vi "Remove.vi"(8 "Error In":errorcluster, 10 "IObserver":refnum<class "IObserver.lvclass">, 11 "reference in":refnum<class "CommunicationModule.lvclass">) -> (0 "Error Out":errorcluster, 3 "reference out":refnum<class "CommunicationModule.lvclass">)   [LabVIEW 2024, in "CommunicationModule.lvclass"]
doc: "Remove observer from the observer list"
uses:
  CommunicationModule.lvclass
  CommunicationModule.lvclass/CommunicationModule.ctl
  IObserver/IObserver.lvclass
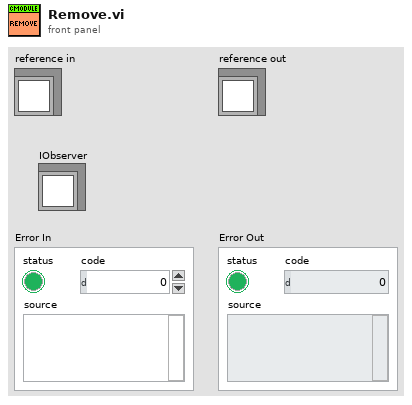
[diagram p1: front panel]
types:
  T1 = typedef "CommunicationModule.lvclass/ObjectAttributes.ctl" = cluster{"ObserverList":refnum<class "IObserver.lvclass">[]}
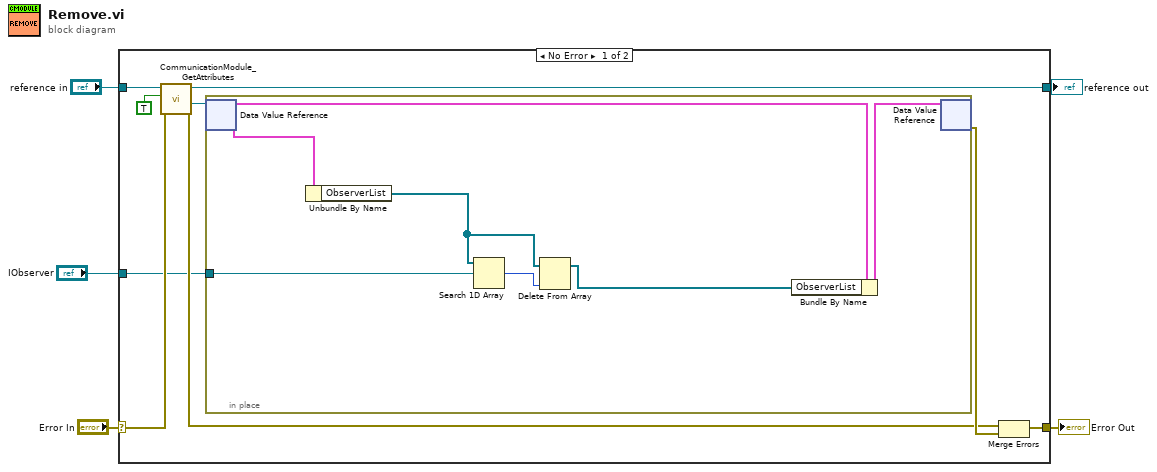
[diagram p0: block diagram]
diagram:
  n1 = case shown="No Error" "Error In" {
    selector: "Error In" -> [w13 w22]
    tunnel: [w10 w22] -> w4
    tunnel: [w11 w21] -> w2
    tunnel: "reference in" -> [w14 w21]
    tunnel: "IObserver" -> [w6 _]
    frame No Error {
      n2 = call "CommunicationModule_GetAttributes.vi"("Error In"=w13, "OnlyGetDvrReference(False)"=TRUE, "reference in"=w14) -> ("Error Out"=w8:errorcluster, "DataRef"=w9:refnum<data-value>, "reference out"=w11:refnum<class "CommunicationModule.lvclass">)  [unwired: 5 in, 1 out]
      n3 = in-place {
        in-place-border: w6 -> [w18]
        n4 = in-place-dvr #1(w9) -> (w19:T1)  [unwired: 1 out]
        n5 = Unbundle By Name(w19) -> ("ObserverList"=w16:refnum<class "IObserver.lvclass">[])
        n6 = Search 1D Array(1D array=w16, element=w18) -> (index of element=w17:i32)  [unwired: 1 in]
        n7 = Delete From Array(array=w16, index=w17) -> (array with subset deleted=w15:refnum<class "IObserver.lvclass">[])  [unwired: 1 in, 1 out]
        n8 = Bundle By Name(cluster=w19, "ObserverList"=w15) -> (w20:T1)
        n9 = in-place-dvr #1(w20) -> (w12:errorcluster)  [unwired: 1 out]
      }
      n10 = Merge Errors(w8, w12) -> (w10:errorcluster)
    }
    frame Error {
    }
  }
  "Error Out" <- w4
  "reference out" <- w2
